vi "Save Item.vi"(8 "error in (no error)":errorcluster, 10 "App Ref":refnum<vi>, 11 "VI in":refnum<class "VI.lvclass">) -> (0 "error out":errorcluster, 2 "Saved?":bool, 3 "VI out":refnum<class "VI.lvclass">)   [LabVIEW 2020, in "VI Properties Editor.lvlib" / "VI.lvclass"]
doc: "Saves the new data of <B>VI in</B>."
uses:
  VI.lvclass
  Control/Control.lvclass
  <vilib>/LabVIEW Icon API/lv_icon/Classes/Icon/Icon.lvclass
  <vilib>/LabVIEW Icon API/LabVIEW Icon API.lvlib
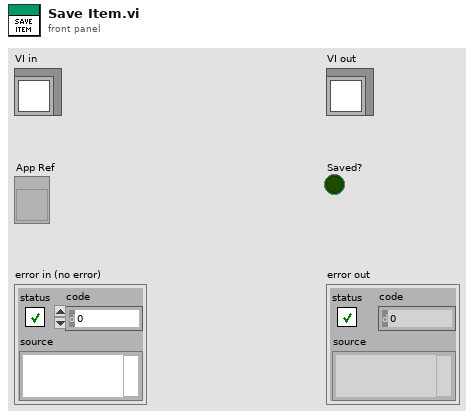
[diagram p1: front panel]
types:
  T1 = enum32{"invalid VI type", "Standard VI", "Control VI", "Global VI", "Polymorphic VI", "Configuration VI", "SubSystem", "Facade VI", "Method VI", "Statechart Diagram VI"}
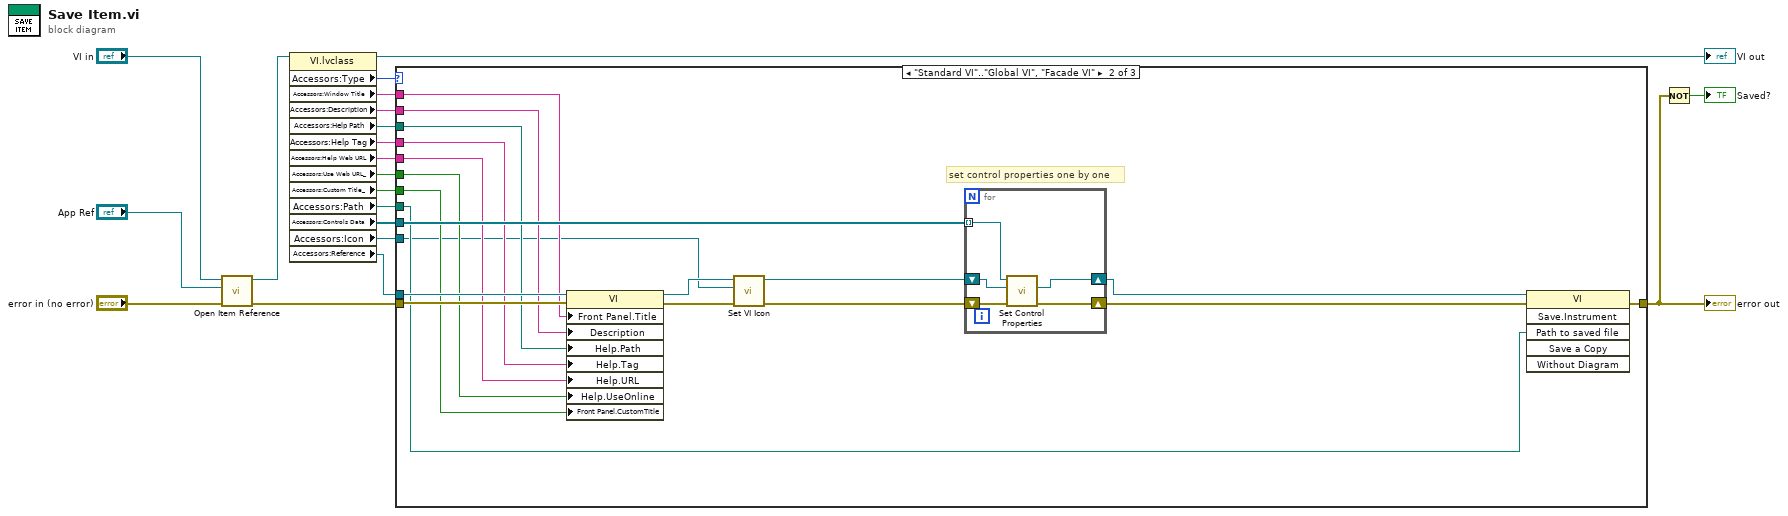
[diagram p0: block diagram]
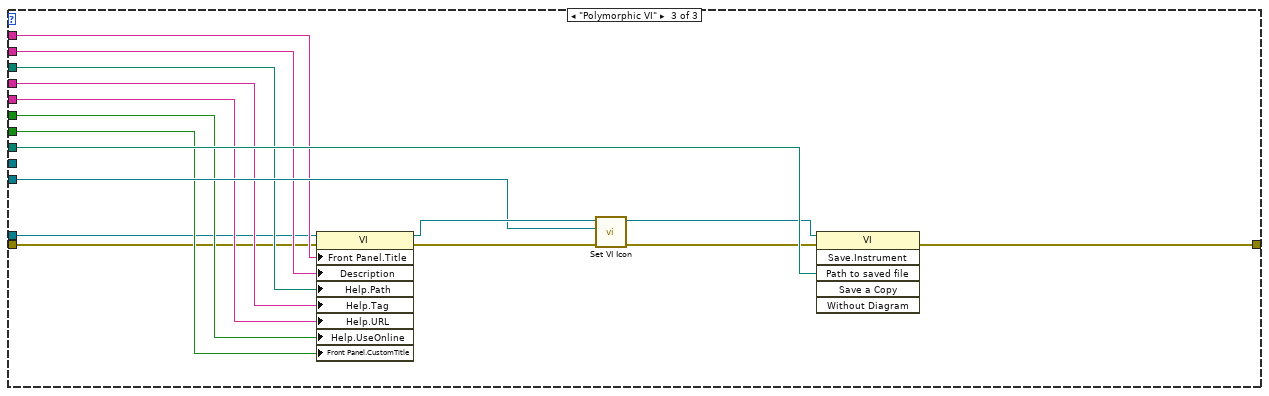
[diagram p3: hidden frame]
diagram:
  n1 = call-dynamic "Open Item Reference.vi"("error in (no error)"="error in (no error)", "App Ref (local)"="App Ref", "VI in"="VI in") -> ("error out"=w18:errorcluster, "VI out"=w15:refnum<class "VI.lvclass">)  [unwired: 7 in]
  n2 = property class="VI.lvclass"(reference=w15) -> (reference out=→"VI out":refnum<class "VI.lvclass">, "Accessors:Type"=w14:T1, "Accessors:Window Title"=w13:string, "Accessors:Description"=w12:string, "Accessors:Help Path"=w11:path, "Accessors:Help Tag"=w10:string, "Accessors:Help Web URL"=w9:string, "Accessors:Use Web URL_"=w8:bool, "Accessors:Custom Title_"=w7:bool, "Accessors:Path"=w6:path, "Accessors:Controls Data"=w5:refnum<class "Control.lvclass">[], "Accessors:Icon"=w2:refnum<class "Icon.lvclass">, "Accessors:Reference"=w4:refnum<vi>)  [unwired: 1 in, 1 out]
  n3 = case shown="\"Standard VI\"..\"Global VI\", \"Facade VI\"" w14 {
    tunnel: [w21 w40 w59] -> w20
    tunnel: w4 -> [_ w36 w48]
    tunnel: w18 -> [w21 w38 w49]
    tunnel: w12 -> [_ w34 w54]
    tunnel: w10 -> [_ w32 w55]
    tunnel: w11 -> [_ w31 w56]
    tunnel: w6 -> [_ w30 w58]
    tunnel: w5 -> [_ w35 _]
    tunnel: w13 -> [_ w33 w53]
    tunnel: w7 -> [_ w29 w57]
    tunnel: w9 -> [_ w28 w52]
    tunnel: w8 -> [_ w27 w51]
    tunnel: w2 -> [_ w25 w60]
    frame "invalid VI type", Default {
    }
    frame "Standard VI".."Global VI", "Facade VI" {
      # "set control properties one by one"
      n4 = property class="VI"(reference=w36, error in=w38, "Front Panel.Title"=w33, "Description"=w34, "Help.Path"=w31, "Help.Tag"=w32, "Help.URL"=w28, "Help.UseOnline"=w27, "Front Panel.CustomTitle"=w29) -> (reference out=w26:refnum<vi>, error out=w37:errorcluster)
      n5 = call <vilib>:"Set VI Icon.vi"("error in (no error)"=w37, "Icon"=w25, "VI Refnum in"=w26) -> ("error out"=w24:errorcluster, "VI Refnum out"=w23:refnum<vi>)  [unwired: 7 in]
      n6 = for {
        shift-right: [w41] -> w39
        shift-left: w24 -> [w45]
        tunnel: w35 -> [w43] mode=indexing
        shift-right: [w42] -> w22
        shift-left: w23 -> [w44]
        n7 = call-dynamic "Set Control Properties.vi"("error in (no error)"=w45, "Owning VI"=w44, "Control in"=w43) -> ("error out"=w41:errorcluster, "dup Owning VI"=w42:refnum<vi>)  [unwired: 6 in, 1 out]
      }
      n8 = invoke class="VI" method="Save.Instrument"(reference=w22, error in=w39, "Path to saved file"=w30) -> (error out=w40:errorcluster)  [unwired: 3 in, 5 out]
    }
    frame "Polymorphic VI" {
      n9 = property class="VI"(reference=w48, error in=w49, "Front Panel.Title"=w53, "Description"=w54, "Help.Path"=w56, "Help.Tag"=w55, "Help.URL"=w52, "Help.UseOnline"=w51, "Front Panel.CustomTitle"=w57) -> (reference out=w61:refnum<vi>, error out=w50:errorcluster)
      n10 = call <vilib>:"Set VI Icon.vi"("error in (no error)"=w50, "Icon"=w60, "VI Refnum in"=w61) -> ("error out"=w47:errorcluster, "VI Refnum out"=w46:refnum<vi>)  [unwired: 7 in]
      n11 = invoke class="VI" method="Save.Instrument"(reference=w46, error in=w47, "Path to saved file"=w58) -> (error out=w59:errorcluster)  [unwired: 3 in, 5 out]
    }
  }
  "error out" <- w20
  n12 = Not(x=w20) -> (.not. x?=→"Saved?":bool)
